vi "index.vi"(0 "二值化图像":T1(plugin-control), 2 "原始图像":T1(plugin-control)) -> (3 "自然形态宽":i32, 4 "自然形态高":i32, 5 "最小外接矩形图":T1(plugin-control), 6 "外接矩形彩色图":T1(plugin-control))   [LabVIEW 2015]
uses:
  <vilib>/vision/NI_Vision_Development_Module.lvlib
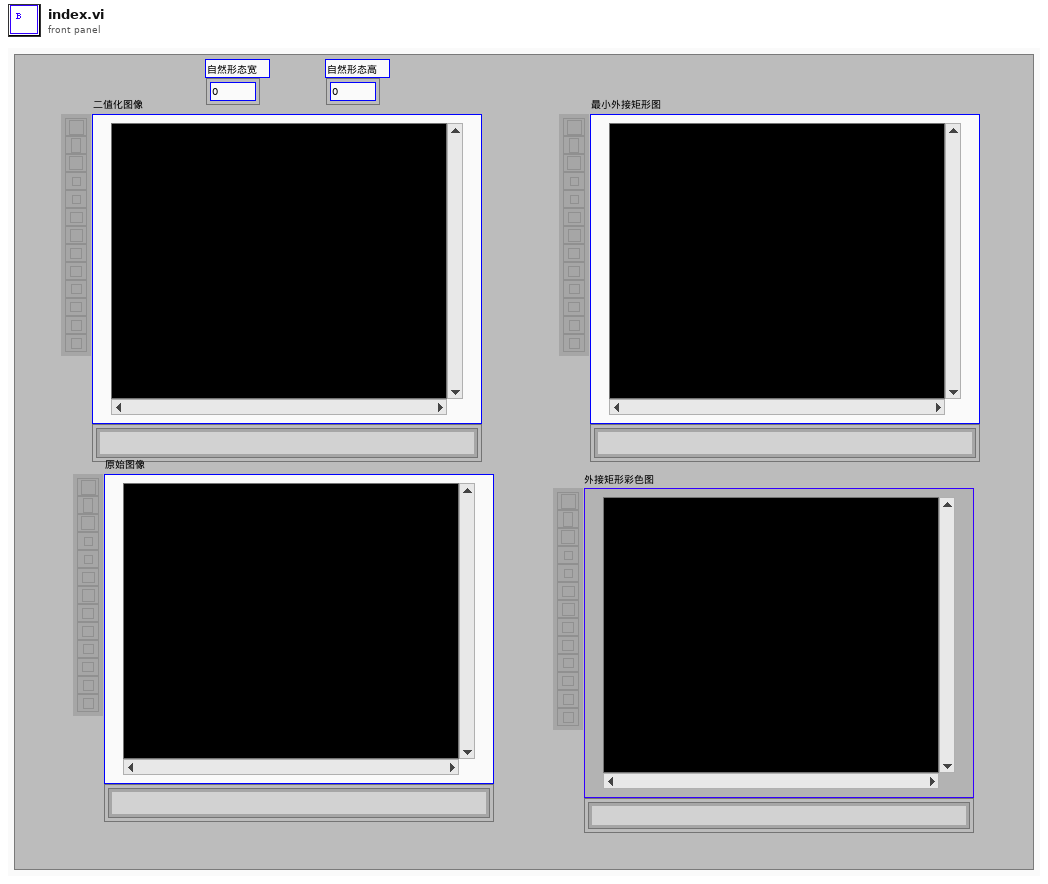
[diagram p1: front panel]
types:
  T1 = typedef "IMAQ Image.ctl" = refnum<image>
  T2 = typedef "Particle Parameters" = i32
  T3 = typedef "Image Type" = u32
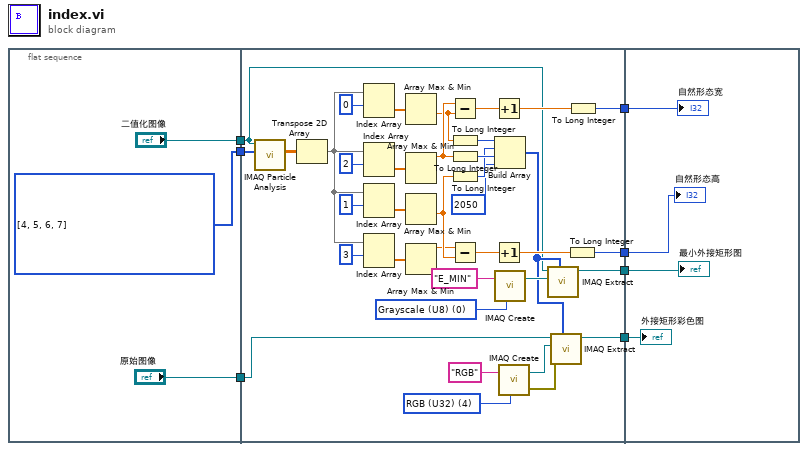
[diagram p0: block diagram]
diagram:
  n1 = flat-sequence {
    tunnel: ["二值化图像"] -> w4
    tunnel: [w9] -> w3
    tunnel: ["原始图像"] -> w2
    tunnel: [w27] -> w7
    tunnel: [w23] -> w6
    tunnel: [w25] -> w5
    tunnel: w4 -> [w16]
    tunnel: w3 -> [w26]
    tunnel: w2 -> [w21]
    tunnel: [w19] -> w1
    tunnel: w7 -> [w51]
    tunnel: w6 -> [w50]
    tunnel: w5 -> [w49]
    tunnel: w1 -> [w48]
    frame #0 {
      w9 = T2[] [4, 5, 6, 7] items=["Center of Mass X", "Center of Mass Y", "First Pixel X", "First Pixel Y", "Bounding Rect Left", "Bounding Rect Top", "Bounding Rect Right", "Bounding Rect Bottom", "Max Feret Diameter Start X", "Max Feret Diameter Start Y", "Max Feret Diameter End X", "Max Feret Diameter End Y", "Max Horiz. Segment Length Left", "Max Horiz. Segment Length Right", "Max Horiz. Segment Length Row", "-", "Bounding Rect Width", "Bounding Rect Height", "Bounding Rect Diagonal", "Perimeter", "Convex Hull Perimeter", "Holes' Perimeter", "Max Feret Diameter", "Equivalent Ellipse Major Axis", "Equivalent Ellipse Minor Axis", "Equivalent Ellipse Minor Axis (Feret)", "Equivalent Rect Long Side", "Equivalent Rect Short Side", "Equivalent Rect Diagonal", "Equivalent Rect Short Side (Feret)", "Average Horiz. Segment Length", "Average Vert. Segment Length", "Hydraulic Radius", "Waddel Disk Diameter", "-", "Area", "Holes' Area", "Particle & Holes' Area", "Convex Hull Area", "Image Area", "-", "Number of Holes", "Number of Horiz. Segments", "Number of Vert. Segments", "-", "Orientation", "Max Feret Diameter Orientation", "-", "% Area/Image Area", "% Area/(Particle & Holes' Area)", "Ratio of Equivalent Ellipse Axes", "Ratio of Equivalent Rect Sides", "-", "Elongation Factor", "Compactness Factor", "Heywood Circularity Factor", "Type Factor", "-", "Sum X", "Sum Y", "Sum XX", "Sum XY", "Sum YY", "Sum XXX", "Sum XXY", "Sum XYY", "Sum YYY", "-", "Moment of Inertia XX", "Moment of Inertia XY", "Moment of Inertia YY", "Moment of Inertia XXX", "Moment of Inertia XXY", "Moment of Inertia XYY", "Moment of Inertia YYY", "Norm. Moment of Inertia XX", "Norm. Moment of Inertia XY", "Norm. Moment of Inertia YY", "Norm. Moment of Inertia XXX", "Norm. Moment of Inertia XXY", "Norm. Moment of Inertia XYY", "Norm. Moment of Inertia YYY", "Hu Moment 1", "Hu Moment 2", "Hu Moment 3", "Hu Moment 4", "Hu Moment 5", "Hu Moment 6", "Hu Moment 7"] ("Pixel Measurements")
    }
    frame #1 {
      w14 = T3 4 items=["Grayscale (U8)", "Grayscale (I16)", "Grayscale (SGL)", "Complex (CSG)", "RGB (U32)", "HSL (U32)", "RGB (U64)", "Grayscale (U16)"] ("Image Type")
      w40 = T3 0 items=["Grayscale (U8)", "Grayscale (I16)", "Grayscale (SGL)", "Complex (CSG)", "RGB (U32)", "HSL (U32)", "RGB (U64)", "Grayscale (U16)"] ("Image Type")
      n2 = call "IMAQ Particle Analysis"("Pixel Measurements"=w26, "Image"=w16) -> ("Particle Measurements (Pixels)"=w28:dbl[][])  [unwired: 3 in, 6 out]
      n3 = Transpose 2D Array(2D array=w28) -> (transposed array=w37:dbl[][])
      n4 = Index Array(array=w37, index (row)=0) -> (element=w35:dbl[])  [unwired: 1 in]
      n5 = Index Array(array=w37, index (row)=2) -> (element=w30:dbl[])  [unwired: 1 in]
      n6 = Index Array(array=w37, index (row)=1) -> (element=w34:dbl[])  [unwired: 1 in]
      n7 = Index Array(array=w37, index (row)=3) -> (element=w31:dbl[])  [unwired: 1 in]
      n8 = Array Max & Min(array=w35) -> (min value=w43:dbl)  [unwired: 3 out]
      n9 = Array Max & Min(array=w30) -> (max value=w46:dbl)  [unwired: 3 out]
      n10 = Array Max & Min(array=w34) -> (min value=w18:dbl)  [unwired: 3 out]
      n11 = Array Max & Min(array=w31) -> (max value=w17:dbl)  [unwired: 3 out]
      n12 = Subtract(x=w46, y=w43) -> (x-y=w38:dbl)
      n13 = To Long Integer(number=w43) -> (32bit integer=w44:i32)
      n14 = To Long Integer(number=w46) -> (32bit integer=w47:i32)
      n15 = To Long Integer(number=w18) -> (32bit integer=w45:i32)
      n16 = Subtract(x=w17, y=w18) -> (x-y=w39:dbl)
      n17 = Increment(x=w38) -> (x+1=w24:dbl)
      n18 = Increment(x=w39) -> (x+1=w22:dbl)
      n19 = Build Array(w44, w45, w47, 2050 ("element")) -> (w20:i32[])
      n20 = call "IMAQ Create"("Image Name"="E_MIN", "Image Type"=w40) -> ("New Image"=w42:T1)  [unwired: 2 in, 2 out]
      n21 = call "IMAQ Create"("Image Name"="RGB", "Image Type"=w14) -> ("New Image"=w12:T1, "error out"=w11:errorcluster)  [unwired: 2 in, 1 out]
      n22 = call "IMAQ Extract"("Optional Rectangle"=w20, "Image Dst"=w42, "Image Src"=w16) -> ("Image Dst Out"=w27:T1)  [unwired: 3 in, 5 out]
      n23 = call "IMAQ Extract"("Optional Rectangle"=w20, "error in (no error)"=w11, "Image Dst"=w12, "Image Src"=w21) -> ("Image Dst Out"=w19:T1)  [unwired: 2 in, 5 out]
      n24 = To Long Integer(number=w22) -> (32bit integer=w23:i32)
      n25 = To Long Integer(number=w24) -> (32bit integer=w25:i32)
    }
    frame #2 {
      "最小外接矩形图" <- w51
      "自然形态高" <- w50
      "自然形态宽" <- w49
      "外接矩形彩色图" <- w48
    }
  }
